vi "User Process Test.vi"() -> ()   [LabVIEW 2014, in "User Control Module Test.lvlib"]
uses:
  User Control Module Test.lvlib
  module/execution/parameter user data.ctl
  module/execution/result user data.ctl
  module/execution/user control module.lvclass
panel:
  in  "stop":bool
  out "error out":errorcluster
  out "Results from processing":T1
  in  "Parameters to process":T2
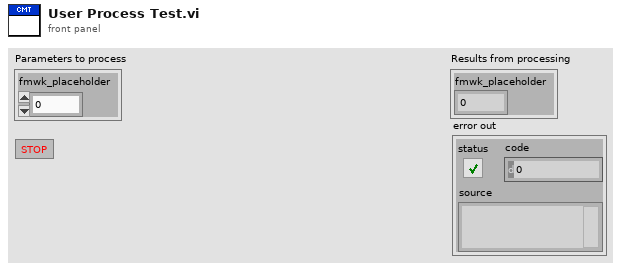
[diagram p1: front panel]
types:
  T1 = typedef "user control module.lvclass/result user data.ctl" = cluster{"fmwk_placeholder":sgl}
  T2 = typedef "user control module.lvclass/parameter user data.ctl" = cluster{"fmwk_placeholder":sgl}
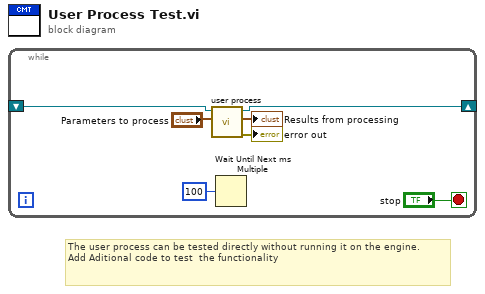
[diagram p0: block diagram]
diagram:
  # "The user process can be tested directly without running it on the engine.\nAdd Aditional code to test  the functionality"
  n1 = while {
    shift-right: [w1] -> _
    shift-left: _ -> [w2]
    stop <- "stop" stop-if-true
    n2 = call "user process.vi"("Parameters to process"="Parameters to process", "user module in"=w2) -> ("error out"=→"error out":errorcluster, "Results from processing"=→"Results from processing":T1, "user module out"=w1:refnum<class "user control module.lvclass">)  [unwired: 7 in]
    n3 = Wait Until Next ms Multiple(millisecond multiple=u32 100) -> ()  [unwired: 1 out]
  }
